vi "Rename Files.vi"(10 "Spec Page Interface":T1, 11 "MetaDataObj in":refnum<class "MetaDataObj.lvclass">) -> (3 "MetaDataObj out":refnum<class "MetaDataObj.lvclass">)   [LabVIEW 2020, in "PluginMetaDataObj.lvclass"]
uses:
  PluginMetaDataObj.lvclass
  <resource>/dialog/NewProjectWizard/Spec Page Interface.ctl
  <resource>/dialog/NewProjectWizard/MetaDataObj/MetaDataObj.lvclass
  C:/Program Files (x86)/National Instruments/LabVIEW 2020/resource/dialog/NewProjectWizard/MetaDataObj/MetaDataObj.lvclass
  <resource>/dialog/NewProjectWizard/MetaDataObj/MetaDataObj.lvclass/MetaDataObj.ctl
  <resource>/dialog/NewProjectWizard/MetaDataObj/Accessors/Write Project Name.vi
  <resource>/dialog/NewProjectWizard/MetaDataObj/Accessors/Write Project Root.vi
  <resource>/dialog/NewProjectWizard/MetaDataObj/Accessors/Write File Prefix.vi
panel:
  in  "Project Name":string
  in  "Project Root":path
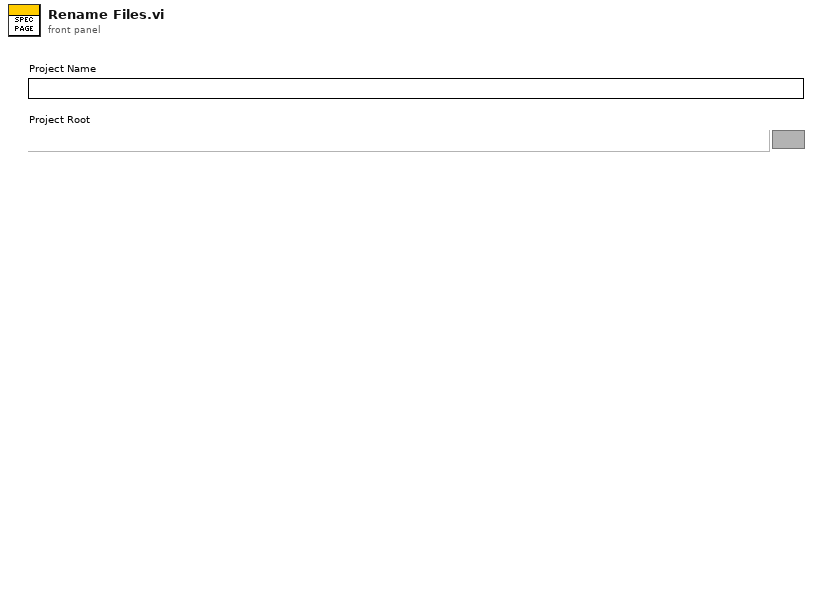
[diagram p1: front panel]
types:
  T1 = typedef "Spec Page Interface.ctl" = cluster{"\"Tab Forward To\" Refnum":refnum<vi>, "\"Tab Backward To\" Refnum":refnum<vi>, "Errors":refnum<user-event>, "Quit":refnum<user-event>}
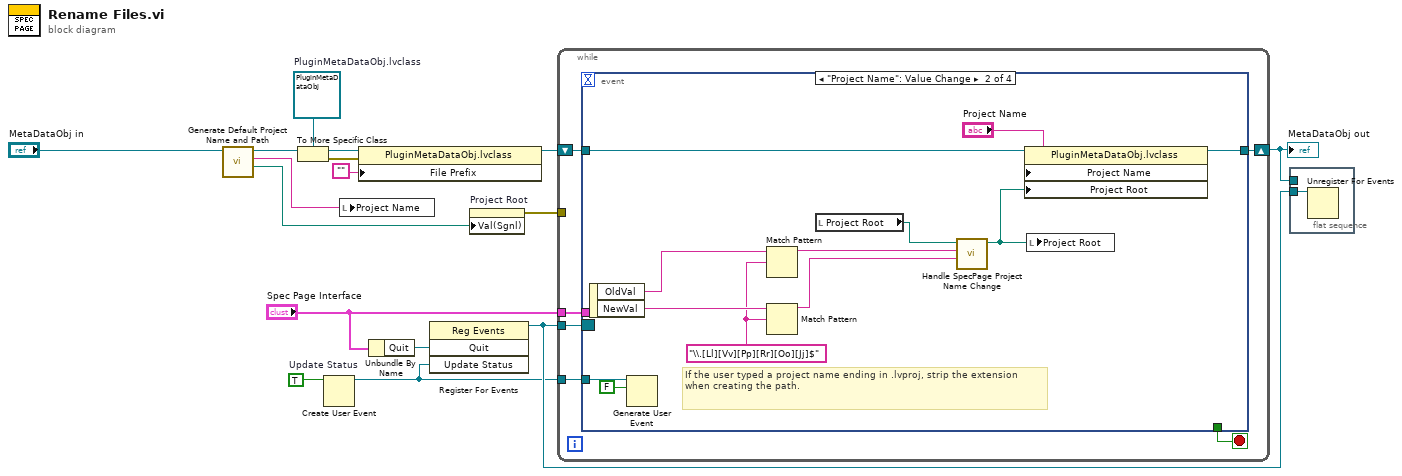
[diagram p0: block diagram]
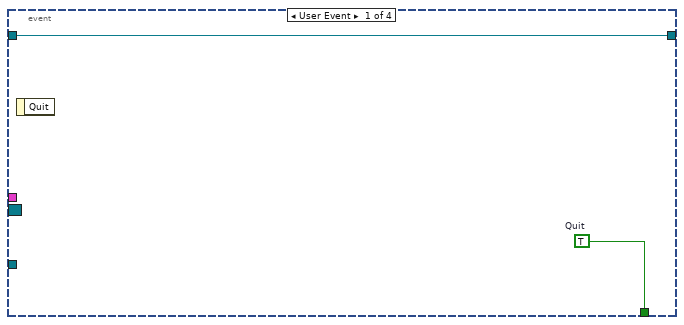
[diagram p2: hidden frame]
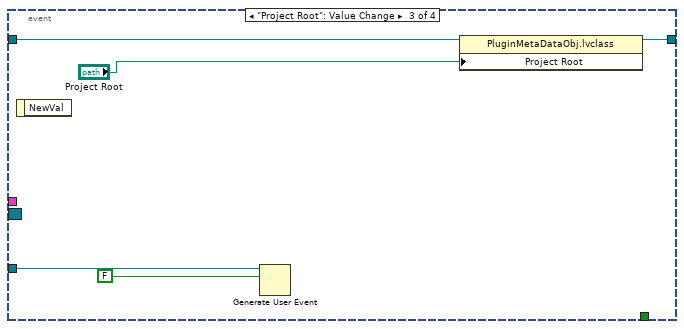
[diagram p3: hidden frame]
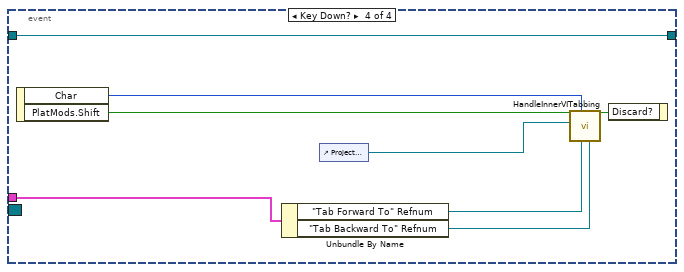
[diagram p4: hidden frame]
diagram:
  w2 = refnum<class "PluginMetaDataObj.lvclass"> refnum  # PluginMetaDataObj.lvclass
  w11 = TRUE  # Update Status
  n1 = call <resource>:"Generate Default Project Name and Path.vi"("DNL_MetaDataObj in"="MetaDataObj in") -> ("Project Root"=w5:path, "Project Name"=w4:string, "DNL_MetaDataObj out"=w6:refnum<class "MetaDataObj.lvclass">)  [unwired: 8 in]
  n2 = To More Specific Class(target class=w2, reference=w6) -> (specific class reference=w13:refnum<class "PluginMetaDataObj.lvclass">, error out=w12:errorcluster)  [unwired: 1 in]
  n3 = Create User Event(user event datatype=w11) -> (user event=w8:refnum<user-event>)  [unwired: 1 in, 1 out]
  n4 = local write "Project Name"(w4) -> ()
  n5 = property class="PluginMetaDataObj.lvclass"(reference=w13, error in=w12, "File Prefix"="") -> (reference out=w10:refnum<class "PluginMetaDataObj.lvclass">)  [unwired: 1 out]
  n6 = Unbundle By Name("Spec Page Interface") -> ("Quit"=w16:refnum<user-event>)
  n7 = register-events(w16, w8) -> (reference out=w15:refnum<event-registration>)  [unwired: 2 in, 1 out]
  n8 = property on="Project Root" class="Path"("Val(Sgnl)"=w5) -> (error out=w9:errorcluster)  [unwired: 2 in, 1 out]
  n9 = while {
    tunnel: "Spec Page Interface" -> [w21]
    shift-right: [w19] -> w1
    shift-left: w10 -> [w18]
    tunnel: w15 -> [w20]
    tunnel: w9 -> [_]
    tunnel: w8 -> [w17]
    stop <- w22 stop-if-true
    n10 = event shown="[1] \"Project Name\": Value Change" {
      selector: w20 -> [_ _ _ _]
      dyn-events: _ -> [_ _ _ _]
      timeout: _ -> [_ _ _ _]
      tunnel: w21 -> [_ _ _ w45]
      tunnel: [w24 _ _ _] -> w22
      tunnel: [w23 w36 w40 w42] -> w19
      tunnel: w18 -> [w23 w33 w41 w42]
      tunnel: w17 -> [_ w35 w39 _]
      event User Event {
        w24 = TRUE  # Quit
        n11 = event-data() -> ()  [unwired: 1 in, 1 out]
      }
      event "Project Name": Value Change {
        w29 = "\\.[Ll][Vv][Pp][Rr][Oo][Jj]$" ("regular expression")
        # "If the user typed a project name ending in .lvproj, strip the extension when creating the path."
        n12 = event-data() -> ("OldVal"=w31:string, "NewVal"=w30:string)  [unwired: 1 in]
        n13 = Generate User Event(user event=w35, event data cluster=FALSE ("Update Status")) -> ()  [unwired: 2 in, 2 out]
        n14 = Match Pattern(string=w31, regular expression=w29) -> (before substring=w28:string)  [unwired: 1 in, 3 out]
        n15 = Match Pattern(string=w30, regular expression=w29) -> (before substring=w27:string)  [unwired: 1 in, 3 out]
        n16 = local read "Project Root"() -> (w32:path)
        n17 = call <resource>:"Handle SpecPage Project Name Change.vi"("Project Name New Value"=w27, "Project Name Old Value"=w28, "Project Root in"=w32) -> ("Project Root out"=w26:path)  [unwired: 8 in]
        n18 = property class="PluginMetaDataObj.lvclass"(reference=w33, "Project Name"="Project Name", "Project Root"=w26) -> (reference out=w36:refnum<class "PluginMetaDataObj.lvclass">)  [unwired: 1 in, 1 out]
        n19 = local write "Project Root"(w26) -> ()
      }
      event "Project Root": Value Change {
        n20 = event-data() -> ()  [unwired: 1 in, 1 out]
        n21 = Generate User Event(user event=w39, event data cluster=FALSE ("Update Status")) -> ()  [unwired: 2 in, 2 out]
        n22 = property class="PluginMetaDataObj.lvclass"(reference=w41, "Project Root"="Project Root") -> (reference out=w40:refnum<class "PluginMetaDataObj.lvclass">)  [unwired: 1 in, 1 out]
      }
      event Key Down? {
        n23 = event-data() -> ("Char"=w48:i16, "PlatMods.Shift"=w47:bool)  [unwired: 1 in]
        n24 = Unbundle By Name(w45) -> ("\"Tab Forward To\" Refnum"=w44:refnum<vi>, "\"Tab Backward To\" Refnum"=w43:refnum<vi>)
        n25 = control-ref of="Project Name"() -> (w46:refnum<vi>)
        n26 = call <resource>:"HandleInnerVITabbing.vi"("Tab Backward To"=w43, "Tab Forward To"=w44, "Char"=w48, "First Control"=w46, "Shift"=w47) -> ("Discard"=w49:bool)  [unwired: 6 in]
        n27 = event-data("Discard?"=w49) -> ()  [unwired: 1 in, 1 out]
      }
    }
  }
  "MetaDataObj out" <- w1
  n28 = flat-sequence {
    tunnel: w15 -> [w50]
    tunnel: w1 -> [_]
    frame #0 {
      n29 = Unregister For Events(event registration refnum=w50) -> ()  [unwired: 1 in, 1 out]
    }
  }
